vi "String as UTF-8 String (UTF-8 String).vi"(9 "error in":errorcluster, 10 "String":refnum<class "UTF-8 String.lvclass">) -> (1 "error out":errorcluster, 2 "UTF-8 String":refnum<class "UTF-8 String.lvclass">)   [LabVIEW 2020, in "G-Unicode.lvlib"]
doc: "Converts the input string to a UTF-8 encoded LabVIEW string."
uses:
  G-Unicode.lvlib
  Types/UTF-8 String/UTF-8 String.lvclass
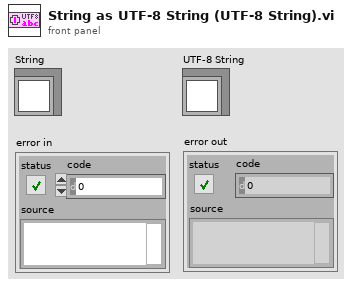
[diagram p1: front panel]
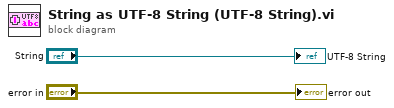
[diagram p0: block diagram]
diagram:
  "UTF-8 String" <- "String"
  "error out" <- "error in"
